vi "Unique Image buffer name - SubVI.vi"(2 "Buffer  base name":string) -> (0 "Image Name":string)   [LabVIEW 2014]
uses:
  Initilize Globals.vi
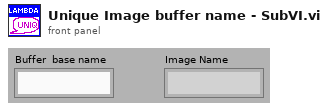
[diagram p1: front panel]
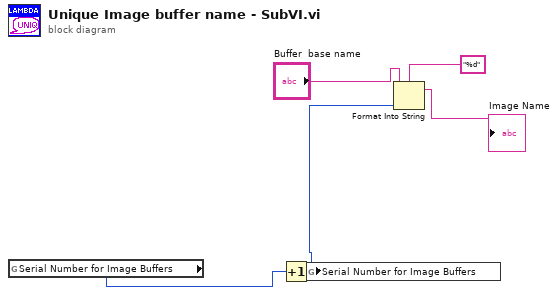
[diagram p0: block diagram]
diagram:
  n1 = global read "Initilize Globals.vi" "Serial Number for Image Buffers"() -> (w2:i32)
  n2 = Increment(x=w2) -> (x+1=w1:i32)
  n3 = global write "Initilize Globals.vi" "Serial Number for Image Buffers"(w1) -> ()
  n4 = Format Into String(format string="%d", initial string="Buffer  base name", w1) -> (resulting string=→"Image Name":string)  [unwired: 1 in, 1 out]
